vi "Update UDP.vi"(8 "error in (no error)":errorcluster, 11 "params":variant) -> (0 "error out":errorcluster)   [LabVIEW 2020]
uses:
  _Controls/Spots.ctl
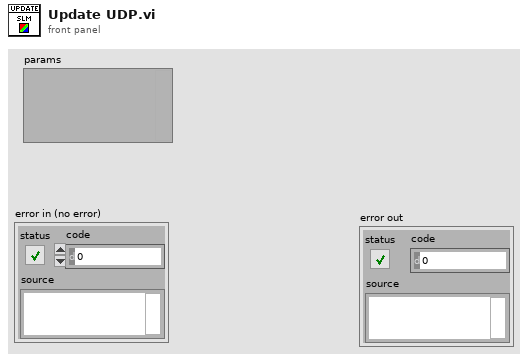
[diagram p1: front panel]
types:
  T1 = typedef "Spots.ctl" = cluster{"Spot Params":cluster{"Intensity":dbl, "Vortex":dbl, "Phase":dbl, "X":dbl, "Y":dbl, "Z":dbl}[], "Add Spot":bool, "Remove Spot":bool, "Clear All Spots":bool, "Save Spots":bool, "Generate Spots":bool, "Generate Spot Pattern":string}
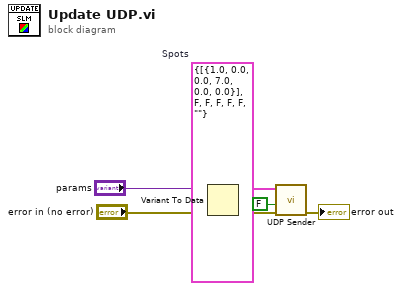
[diagram p0: block diagram]
diagram:
  w4 = T1 {"Spot Params"=[{"Intensity"=1.0, "Vortex"=0.0, "Phase"=0.0, "X"=7.0, "Y"=0.0, "Z"=0.0}], "Add Spot"=FALSE, "Remove Spot"=FALSE, "Clear All Spots"=FALSE, "Save Spots"=FALSE, "Generate Spots"=FALSE, "Generate Spot Pattern"=""}  # Spots
  n1 = Variant To Data(error in="error in (no error)", type=w4, Variant="params") -> (data=w1:T1, error out=w3:errorcluster)
  n2 = call "UDP Sender.vi"("error in"=w3, "Show panel"=FALSE, "Spots"=w1) -> ("error out"=→"error out":errorcluster)  [unwired: 3 in, 1 out]
